vi "InitPostions (SubVI).vi"(11 "ControlCluster":T1) -> ()   [LabVIEW 2022 SP3]
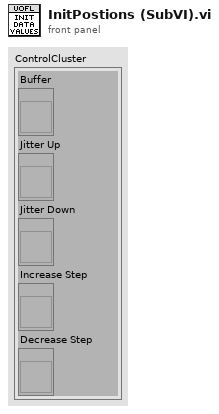
[diagram p1: front panel]
types:
  T1 = cluster{"Buffer":refnum<vi>, "Jitter Up":refnum<vi>, "Jitter Down":refnum<vi>, "Increase Step":refnum<vi>, "Decrease Step":refnum<vi>}
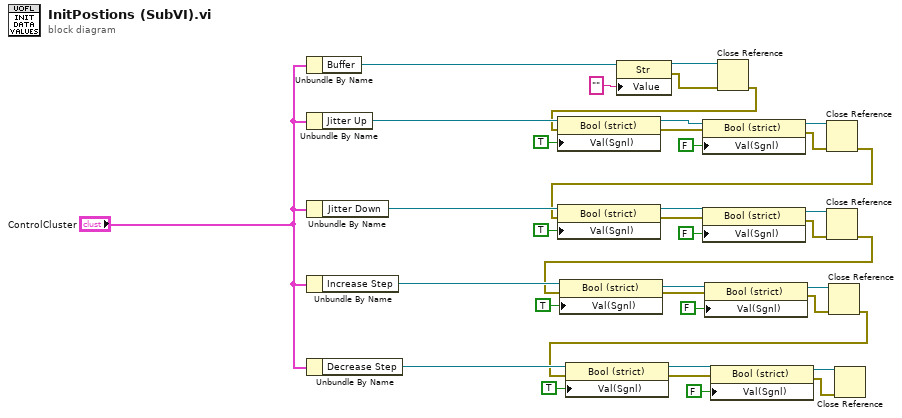
[diagram p0: block diagram]
diagram:
  n1 = Unbundle By Name("ControlCluster") -> ("Buffer"=w27:refnum<vi>)
  n2 = Unbundle By Name("ControlCluster") -> ("Jitter Up"=w28:refnum<vi>)
  n3 = Unbundle By Name("ControlCluster") -> ("Jitter Down"=w12:refnum<vi>)
  n4 = Unbundle By Name("ControlCluster") -> ("Increase Step"=w7:refnum<vi>)
  n5 = Unbundle By Name("ControlCluster") -> ("Decrease Step"=w6:refnum<vi>)
  n6 = property on="Property Node" class="Str"(reference=w27, "Value"="") -> (reference out=w36:refnum<vi>, error out=w37:errorcluster)  [unwired: 1 in]
  n7 = Close Reference(reference=w36, error in (no error)=w37) -> (error out=w13:errorcluster)
  n8 = property on="Property Node" class="Bool (strict)"(reference=w28, error in=w13, "Val(Sgnl)"=TRUE ("Value (Signaling)")) -> (reference out=w32:refnum<vi>, error out=w31:errorcluster)
  n9 = property on="Property Node" class="Bool (strict)"(reference=w32, error in=w31, "Val(Sgnl)"=FALSE ("Value (Signaling)")) -> (reference out=w33:refnum<vi>, error out=w34:errorcluster)
  n10 = Close Reference(reference=w33, error in (no error)=w34) -> (error out=w3:errorcluster)
  n11 = property on="Property Node" class="Bool (strict)"(reference=w12, error in=w3, "Val(Sgnl)"=TRUE ("Value (Signaling)")) -> (reference out=w11:refnum<vi>, error out=w24:errorcluster)
  n12 = property on="Property Node" class="Bool (strict)"(reference=w11, error in=w24, "Val(Sgnl)"=FALSE ("Value (Signaling)")) -> (reference out=w10:refnum<vi>, error out=w23:errorcluster)
  n13 = Close Reference(reference=w10, error in (no error)=w23) -> (error out=w2:errorcluster)
  n14 = property on="Property Node" class="Bool (strict)"(reference=w7, error in=w2, "Val(Sgnl)"=TRUE ("Value (Signaling)")) -> (reference out=w8:refnum<vi>, error out=w21:errorcluster)
  n15 = property on="Property Node" class="Bool (strict)"(reference=w8, error in=w21, "Val(Sgnl)"=FALSE ("Value (Signaling)")) -> (reference out=w9:refnum<vi>, error out=w22:errorcluster)
  n16 = Close Reference(reference=w9, error in (no error)=w22) -> (error out=w1:errorcluster)
  n17 = property on="Property Node" class="Bool (strict)"(reference=w6, error in=w1, "Val(Sgnl)"=TRUE ("Value (Signaling)")) -> (reference out=w5:refnum<vi>, error out=w16:errorcluster)
  n18 = property on="Property Node" class="Bool (strict)"(reference=w5, error in=w16, "Val(Sgnl)"=FALSE ("Value (Signaling)")) -> (reference out=w4:refnum<vi>, error out=w15:errorcluster)
  n19 = Close Reference(reference=w4, error in (no error)=w15) -> ()  [unwired: 1 out]
